vi "Digital - Continuous Output.vi"() -> ()   [LabVIEW 2012]
doc: "This example demonstrates how to generate a continuous amount of digital data based off of a sample clock.\n\nSome hardware (e.g. M Series DAQ) must use an external sample clock for digital tasks. To view a complete list of available sample clock sources, consult the Device Routes table in Measurement and Automation Explorer.\n\nFor instructions on how to connect your signals to the DAQ device, refer to your device documentation."
uses:
  <vilib>/DAQmx/write.llb/DAQmx Write (Digital 1D U32 1Chan NSamp).vi
  <vilib>/DAQmx/create/channels.llb/DAQmx Create Channel (DO-Digital Output).vi
  <vilib>/DAQmx/configure/timing.llb/DAQmx Timing (Sample Clock).vi
  <vilib>/DAQmx/configure/trigger.llb/DAQmx Start Trigger (Digital Edge).vi
  <vilib>/DAQmx/miscellaneous.llb/DAQmx Fill In Error Info.vi
  <resource>/objmgr/daqmx.rc
panel:
  in  "Line(s)":tag="Dev1/port0/line0:7"
  in  "Stop":bool
  in  "Output Array":u32[](array[numeric])=[1, 2, 4, 8, 16, 32, 64, 128]
  in  "Trigger Type":enum32{"No Trigger", "Digital Start"}(tab)
  in  "Edge":i32(ring)=10280 items=["Rising"=10280, "Falling"=10171]
  in  "Digital Trigger Source":tag="PFI1"
  in  "Number of Samples":i32=1000
  in  "Sample Rate":dbl=1000.0
  in  "Sample Clock Source":tag="PFI0"
  out "Actual Sample Rate":dbl=1000.0 format="%0.2f"
  # "Channel Settings"
  # "Data to Write"
  # "Timing and Buffer Settings"
  # "Trigger Settings"
  # "To configure and use a start trigger you must have the necessary tab selected above.  Not all hardware supports triggering--refer to your device documentation for more info."
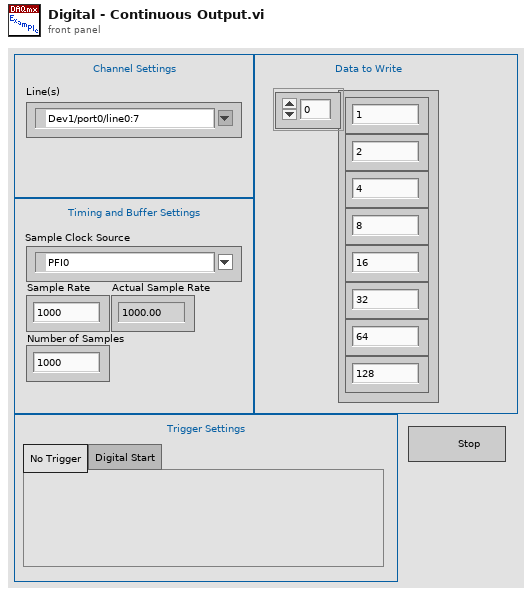
[diagram p1: front panel]
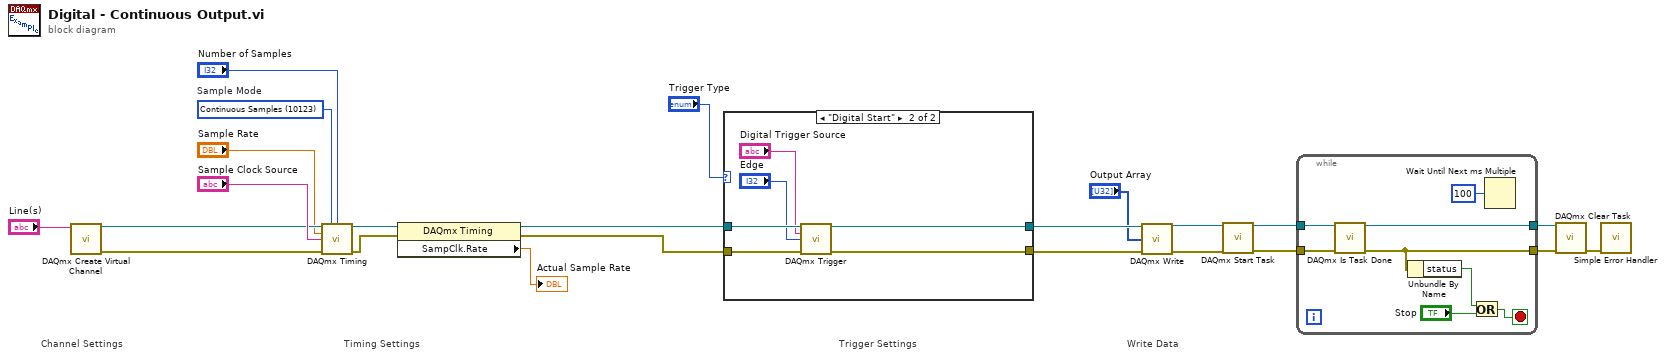
[diagram p0: block diagram]
diagram:
  w16 = 10123 items=["Finite Samples"=10178, "Continuous Samples"=10123, "Hardware Timed Single Point"=12522]  # Sample Mode
  # "Trigger Settings"
  # "Timing Settings"
  # "Write Data"
  # "Channel Settings"
  n1 = call-poly <vilib>:"DAQmx Create Virtual Channel.vi"("lines"="Line(s)") -> ("task out"=w20:refnum<k21>, "error out"=w19:errorcluster)  [unwired: 13 in]
  n2 = call-poly <vilib>:"DAQmx Timing.vi"("task/channels in"=w20, "sample mode"=w16, "samples per channel"="Number of Samples", "rate"="Sample Rate", "source"="Sample Clock Source", "error in"=w19) -> ("task out"=w15:refnum<k21>, "error out"=w14:errorcluster)  [unwired: 8 in]
  n3 = property class="DAQmx Timing"(reference=w15, error in=w14) -> (reference out=w12:refnum<k21>, error out=w11:errorcluster, "SampClk.Rate"=→"Actual Sample Rate":dbl)
  n4 = case shown="\"Digital Start\"" "Trigger Type" {
    tunnel: w12 -> [w25 w31]
    tunnel: w11 -> [w24 w30]
    tunnel: [w25 w29] -> w10
    tunnel: [w24 w28] -> w9
    frame "No Trigger", Default {
    }
    frame "Digital Start" {
      n5 = call-poly <vilib>:"DAQmx Trigger.vi"("task/channels in"=w31, "source"="Digital Trigger Source", "edge"="Edge", "error in"=w30) -> ("task out"=w29:refnum<k21>, "error out"=w28:errorcluster)  [unwired: 10 in]
    }
  }
  n6 = call-poly <vilib>:"DAQmx Write.vi"("task/channels in"=w10, "data"="Output Array", "error in"=w9) -> ("task out"=w7:refnum<k21>, "error out"=w6:errorcluster)  [unwired: 10 in, 1 out]
  n7 = call <vilib>:"DAQmx Start Task.vi"("task/channels in"=w7, "error in"=w6) -> ("task out"=w5:refnum<k21>, "error out"=w4:errorcluster)  [unwired: 12 in]
  n8 = while {
    tunnel: w5 -> [w39]
    tunnel: w4 -> [w38]
    tunnel: [w35] -> w3
    tunnel: [w37] -> w2
    stop <- w32 stop-if-true
    n9 = call <vilib>:"DAQmx Is Task Done.vi"("task/channels in"=w39, "error in"=w38) -> ("task out"=w37:refnum<k21>, "error out"=w35:errorcluster)  [unwired: 11 in, 1 out]
    n10 = Unbundle By Name(w35) -> ("status"=w34:bool)
    n11 = Or(x=w34, y="Stop") -> (x .or. y?=w32:bool)
    n12 = Wait Until Next ms Multiple(millisecond multiple=u32 100) -> ()  [unwired: 1 out]
  }
  n13 = call <vilib>:"DAQmx Clear Task.vi"("task in"=w2, "error in"=w3) -> ("error out"=w23:errorcluster)  [unwired: 13 in]
  n14 = call <vilib>:"Simple Error Handler.vi"("error in (no error)"=w23) -> ()  [unwired: 4 in, 5 out]
